vi "DriverFEFY6900.vi"() -> ()   [LabVIEW 2024]
uses:
  <vilib>/Instr/_visa.llb/VISA Set IO Buffer Mask.ctl
  <vilib>/Instr/_visa.llb/VISA Flush IO Buffer Mask.ctl
  <vilib>/Instr/_visa.llb/VISA Configure Serial Port (Instr).vi
panel:
  in  "Parametres":T1
  out "IDnumber":string="COM6"
  in  "Channel A OnOff":bool
  in  "AM FM PM":string[](array[string])=["ChannelB", "Ext VCO - IN"]
  in  "FSK ASK PSK BURS":string[](array[string])=["ChannelB", "Ext AC", "Manual", "Ext DC"]
  out "ChannelB\nChannelBState":bool
  in  "ChannelB OnOff":bool
  in  "Channel B":T2 {"Frequence" min=0.0 max=60000000.0 step=10000000.0 scale=0.0..60000000.0 scale format="%#_6p"; "Phase" scale=0.0..360.0; "DutyCycle" scale=0.0..100.0; "Offset" min=-12.0 max=12.0 step=1.0; "Amplitude" min=0.0 max=24.0 step=1.0}
  out "ChannelAState":bool
  in  "Channel A":T3={"WaveForme"=enum."Sine", "Amplitude"=0.0, "Offset"=0.0, "DutyCycle"=0.0, "Phase"=0.0, "Frequence"=0.0, "Modulation mode"=enum."FSK", "Modulation source"=0, "Trigger Pulse"=0, "FSK frequence"=0, "Manual Sources"=FALSE, " AM modu rate"=0.0, "FM Freq offset"=1000000.0, " PM modu offset"=0.0, "Sweep mode"=enum."Frequency", "Sweep start"=0.0, "Sweep end"=0.0, "Sweep Time (sec)"=0.01, "Type Sweep"=enum."Linear", "Sweep ON/OFF"=FALSE, "Source sweep"=enum."Time", "Incr"=enum."1uHz", "Incr FSK"=enum."1uHz", "Incr Trigger"=enum."1u", "Incr FM"=enum."1uHz"} {"Sweep Time (sec)" min=0.01 max=1000.0 step=1.0 scale=0.0..1000.0; "Sweep end" scale=-12.0..12.0 scale format="%#_6p"; "Sweep start" scale=-12.0..12.0 scale format="%#_6p"; "PM modu offset" min=0.0 max=360.0 step=1.0 scale=0.0..360.0; "FM Freq offset" max=60000000.0 step=1e-06 scale=0.0..60000000.0 scale format="%#_1p"; "AM modu rate" scale=0.0..100.0; "FSK frequence" max=60000000 step=1 scale=0.0..60000000.0 scale format="%.1p"; "Trigger Pulse" max=1048575 step=100 scale=0.0..1048575.0 scale format="%.1p"; "Modulation source" items=["ChannelB", "Ext AC", "Manual", "Ext DC"]; "Frequence" min=0.0 max=60000000.0 step=1e-06 scale=0.0..60000000.0 scale format="%#_6p"; "Phase" scale=0.0..360.0; "DutyCycle" scale=0.0..100.0; "Offset" min=-12.0 max=12.0 step=1.0; "Amplitude" min=0.0 max=24.0 step=1.0}
  out "Com":bool
  in  "PortCOM":string="COM6"
  in  "stop":bool
  in  "Enable Termination\nChar (T)":bool=TRUE
  # "PORT COM"
  # "Sauvegardes et paramètres"
  # "Sweep"
  # "Modulation - Trigger"
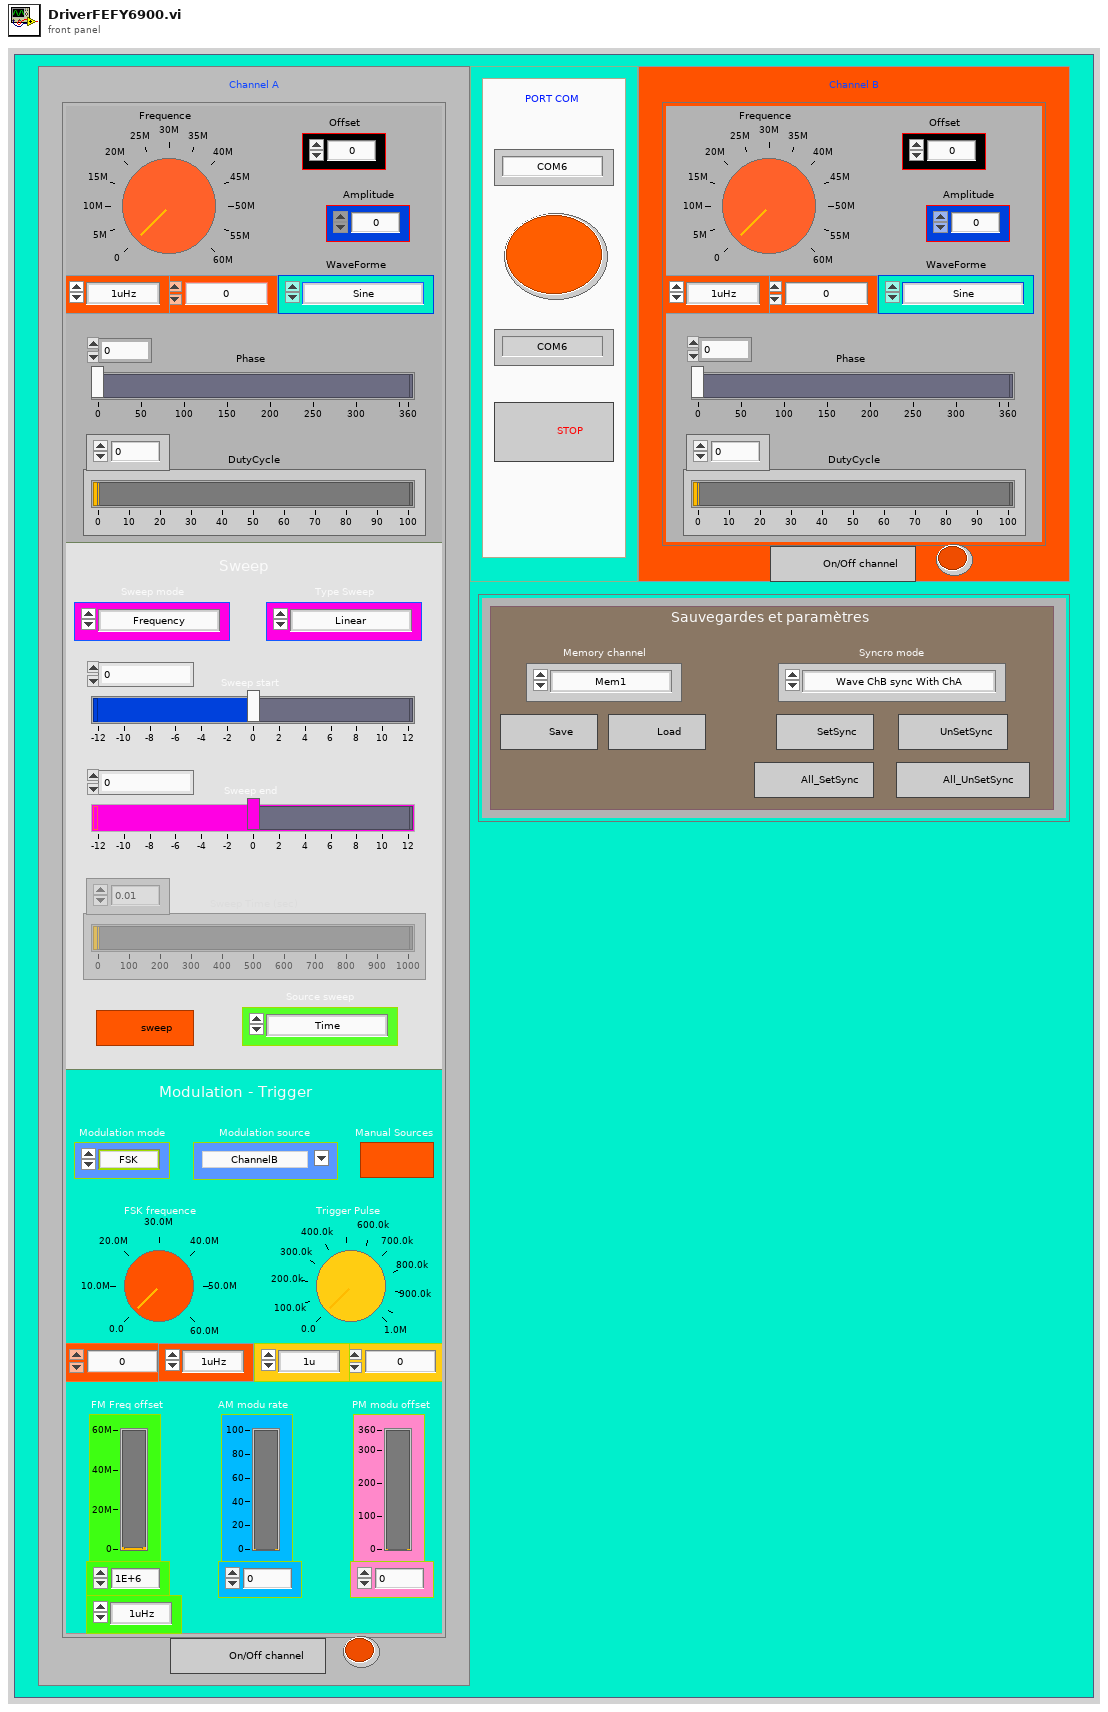
[diagram p1: front panel]
types:
  T1 = cluster{"Memory channel":enum16{"Mem1", "Mem2", "Mem3", "Mem4", "Mem5", "Mem6"}, "Save All param":bool, "Load param":bool, "Syncro mode":enum16{"Wave ChB sync With ChA", "Freq ChB sync With ChA ", "Ampli ChB sync With ChA", "Offset ChB sync With ChA", "DutyC ChB sync With ChA"}, "Set Sync":bool, "UnSet Sync":bool, "All Set Sync":bool, "All UnSet Sync":bool}
  T2 = cluster{"WaveForme":enum16{"Sine", "Square", "Rectangle", "Trapezoid1", "Cmos", "DC", "Triangle", "RAMP", "NegRAMP", "Stair_Triangle", "Stair_Step", "Neg_Stair", "Pos_Exponen", "Neg_Exponen", "P_Fall_Exp", "N_Fall_Exp", "PosLogarit", "NegLogarit", "P_Fall_Log", "N_Fall_Log", "P_Full_Wav", "N_Full_Wav", "P_Half_Wav", "N_Half_Wav", "LorentzPU", "Multitone", "Random_Noise", "ECG", "Trapezoid2", "Sinc_Pulse", "Impulse1", "AWGN", "AM", "FM", "Chrip", "Impulse2", "Arbitraire1", "Arbitraire2"}, "Amplitude":dbl, "Offset":dbl, "DutyCycle":dbl, "Phase":dbl, "Frequence":dbl, "Incr":enum16{"1uHz", "10uHz", "100uHz", "1mHz", "10mHz", "100mHz", "1Hz", "10Hz", "100Hz", "1Khz", "10Khz", "100Khz", "1Mhz", "10Mhz"}}
  T3 = cluster{"WaveForme":enum16{"Sine", "Square", "Rectangle", "Trapezoid1", "Cmos", "ADJ_PULSE", "DC", "Triangle", "RAMP", "NegRAMP", "Stair_Triangle", "Stair_Step", "Neg_Stair", "Pos_Exponen", "Neg_Exponen", "P_Fall_Exp", "N_Fall_Exp", "PosLogarit", "NegLogarit", "P_Fall_Log", "N_Fall_Log", "P_Full_Wav", "N_Full_Wav", "P_Half_Wav", "N_Half_Wav", "LorentzPU", "Multitone", "Random_Noise", "ECG", "Trapezoid2", "Sinc_Pulse", "Impulse1", "AWGN", "AM", "FM", "Chrip", "Impulse2", "Arbitraire1", "Arbitraire2"}, "Amplitude":dbl, "Offset":dbl, "DutyCycle":dbl, "Phase":dbl, "Frequence":dbl, "Modulation mode":enum16{"FSK", "ASK", "PSK", "Burs", "AM", "FM", "PM"}, "Modulation source":u16, "Trigger Pulse":u32, "FSK frequence":u32, "Manual Sources":bool, " AM modu rate":dbl, "FM Freq offset":dbl, " PM modu offset":dbl, "Sweep mode":enum16{"Frequency", "Amplitude", "Offset", "DutyCycle"}, "Sweep start":dbl, "Sweep end":dbl, "Sweep Time (sec)":dbl, "Type Sweep":enum16{"Linear", "Logarithm"}, "Sweep ON/OFF":bool, "Source sweep":enum16{"Time", "VCO IN"}, "Incr":enum16{"1uHz", "10uHz", "100uHz", "1mHz", "10mHz", "100mHz", "1Hz", "10Hz", "100Hz", "1Khz", "10Khz", "100Khz", "1Mhz", "10Mhz"}, "Incr FSK":enum16{"1uHz", "10uHz", "100uHz", "1mHz", "10mHz", "100mHz", "1Hz", "10Hz", "100Hz", "1Khz", "10Khz", "100Khz", "1Mhz", "10Mhz"}, "Incr Trigger":enum16{"1u", "10u", "100u", "1m", "10m", "100m", "1", "10", "100", "1K", "10K", "100K"}, "Incr FM":enum16{"1uHz", "10uHz", "100uHz", "1mHz", "10mHz", "100mHz", "1Hz", "10Hz", "100Hz", "1Khz", "10Khz", "100Khz", "1Mhz", "10Mhz"}}
  T4 = typedef "VISA Set IO Buffer Mask.ctl" = u16
  T5 = enum8{"Enabled", "Disabled", "Disabled and Grayed Out"}
  T6 = enum16{"Sine", "Square", "Rectangle", "Trapezoid1", "Cmos", "ADJ_PULSE", "DC", "Triangle", "RAMP", "NegRAMP", "Stair_Triangle", "Stair_Step", "Neg_Stair", "Pos_Exponen", "Neg_Exponen", "P_Fall_Exp", "N_Fall_Exp", "PosLogarit", "NegLogarit", "P_Fall_Log", "N_Fall_Log", "P_Full_Wav", "N_Full_Wav", "P_Half_Wav", "N_Half_Wav", "LorentzPU", "Multitone", "Random_Noise", "ECG", "Trapezoid2", "Sinc_Pulse", "Impulse1", "AWGN", "AM", "FM", "Chrip", "Impulse2", "Arbitraire1", "Arbitraire2"}
  T7 = typedef "VISA Flush IO Buffer Mask.ctl" = u16
  T8 = enum16{"FSK", "ASK", "PSK", "Burs", "AM", "FM", "PM"}
  T9 = enum16{"Sine", "Square", "Rectangle", "Trapezoid1", "Cmos", "DC", "Triangle", "RAMP", "NegRAMP", "Stair_Triangle", "Stair_Step", "Neg_Stair", "Pos_Exponen", "Neg_Exponen", "P_Fall_Exp", "N_Fall_Exp", "PosLogarit", "NegLogarit", "P_Fall_Log", "N_Fall_Log", "P_Full_Wav", "N_Full_Wav", "P_Half_Wav", "N_Half_Wav", "LorentzPU", "Multitone", "Random_Noise", "ECG", "Trapezoid2", "Sinc_Pulse", "Impulse1", "AWGN", "AM", "FM", "Chrip", "Impulse2", "Arbitraire1", "Arbitraire2"}
  T10 = enum16{"Mem1", "Mem2", "Mem3", "Mem4", "Mem5", "Mem6"}
  T11 = enum16{"Wave ChB sync With ChA", "Freq ChB sync With ChA ", "Ampli ChB sync With ChA", "Offset ChB sync With ChA", "DutyC ChB sync With ChA"}
  T12 = enum16{"Frequency", "Amplitude", "Offset", "DutyCycle"}
  T13 = enum16{"1uHz", "10uHz", "100uHz", "1mHz", "10mHz", "100mHz", "1Hz", "10Hz", "100Hz", "1Khz", "10Khz", "100Khz", "1Mhz", "10Mhz"}
  T14 = enum16{"1u", "10u", "100u", "1m", "10m", "100m", "1", "10", "100", "1K", "10K", "100K"}
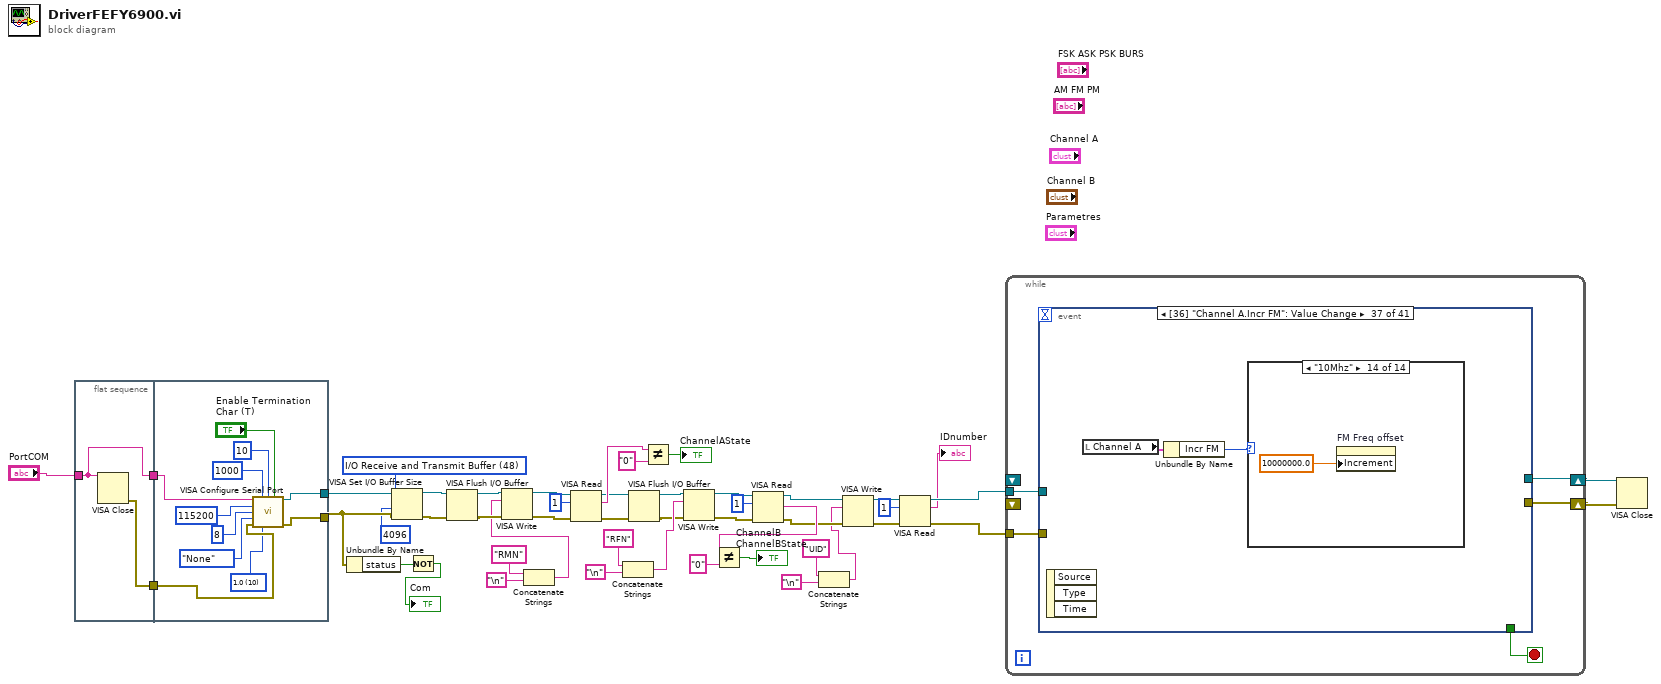
[diagram p0: block diagram]
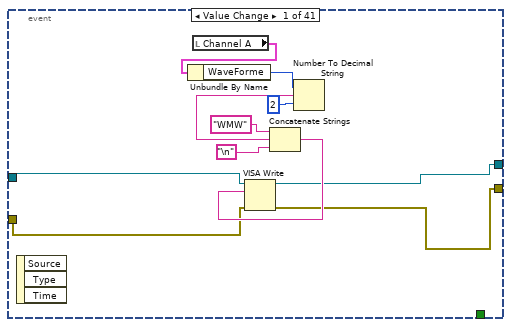
[diagram p2: hidden frame]
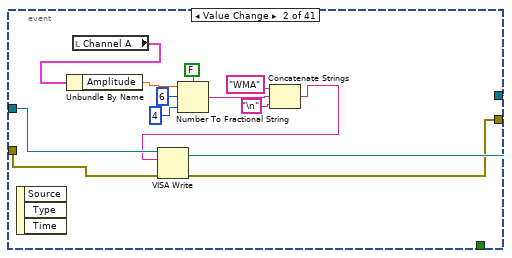
[diagram p3: hidden frame]
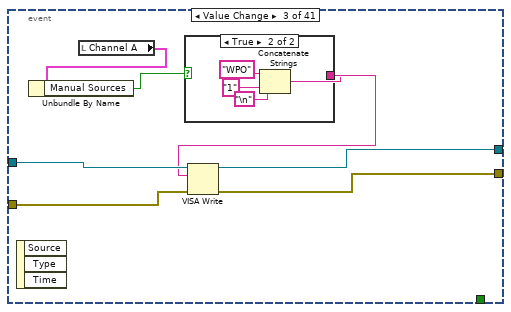
[diagram p4: hidden frame]
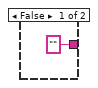
[diagram p5: hidden frame]
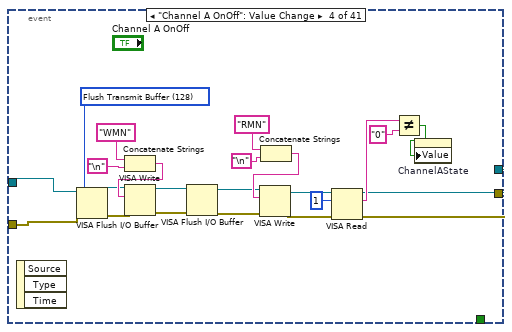
[diagram p6: hidden frame]
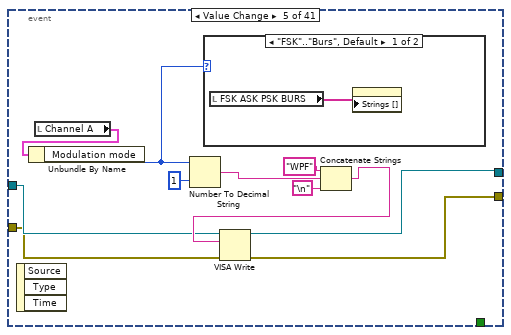
[diagram p7: hidden frame]
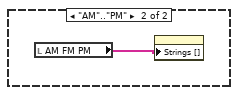
[diagram p8: hidden frame]
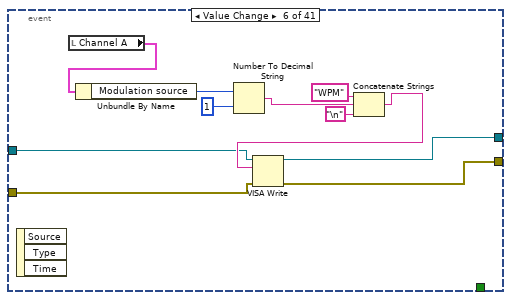
[diagram p9: hidden frame]
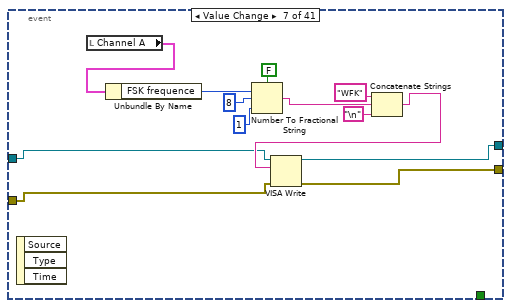
[diagram p10: hidden frame]
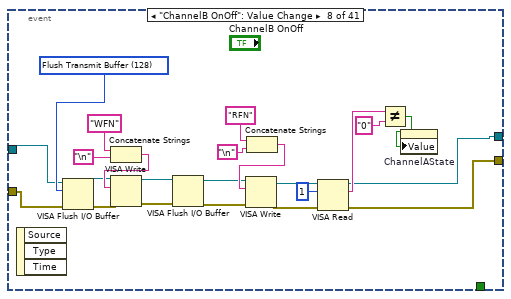
[diagram p11: hidden frame]
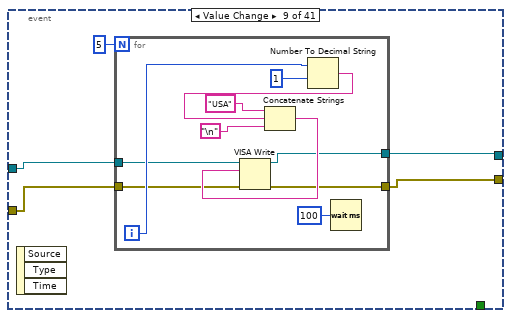
[diagram p12: hidden frame]
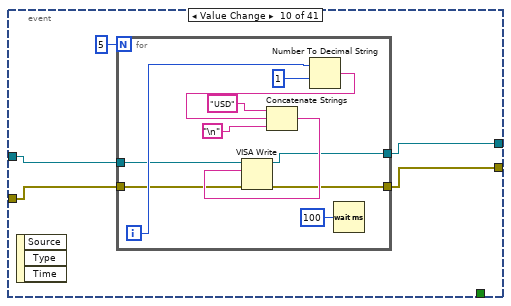
[diagram p13: hidden frame]
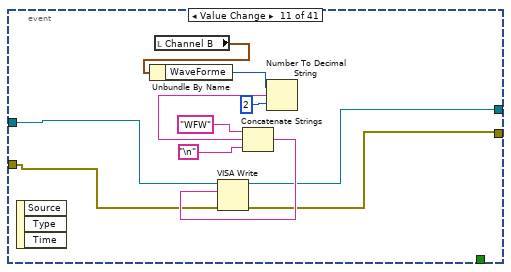
[diagram p14: hidden frame]
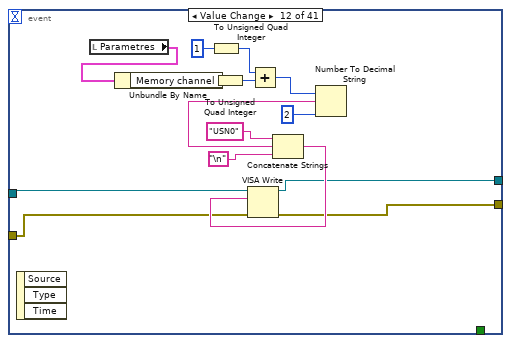
[diagram p15: hidden frame]
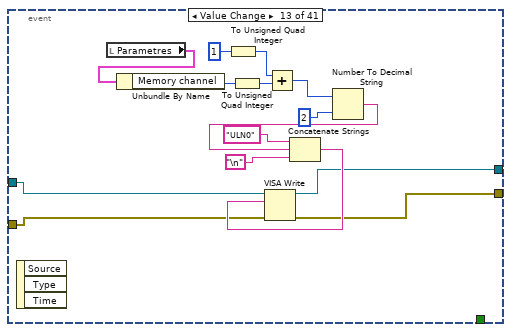
[diagram p16: hidden frame]
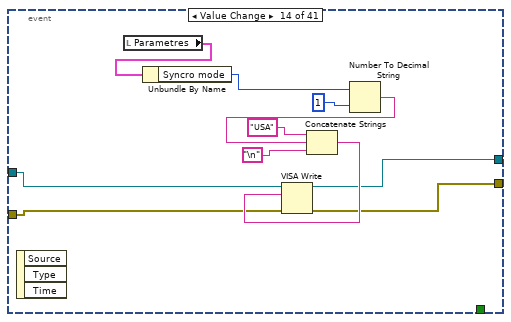
[diagram p17: hidden frame]
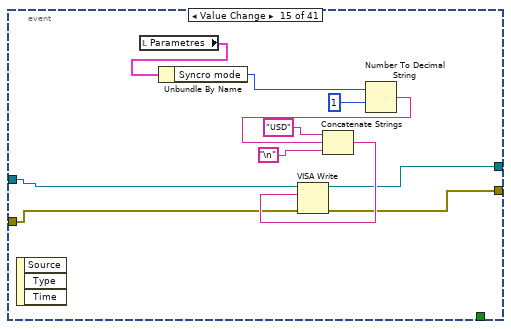
[diagram p18: hidden frame]
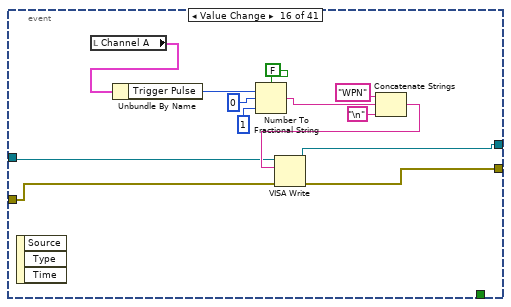
[diagram p19: hidden frame]
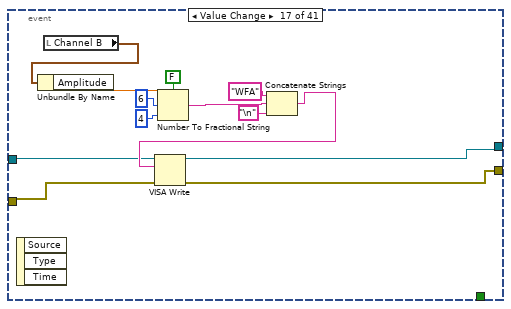
[diagram p20: hidden frame]
diagram:
  w38 = T4 48 items=["I/O Receive Buffer"=16, "I/O Transmit Buffer"=32, "I/O Receive and Transmit Buffer"=48] ("Mask")
  n1 = flat-sequence {
    tunnel: "PortCOM" -> [w50]
    tunnel: [w50] -> w45
    tunnel: [w49] -> w44
    tunnel: w45 -> [w60]
    tunnel: w44 -> [w54]
    tunnel: [w52] -> w41
    tunnel: [w51] -> w40
    frame #0 {
      n2 = VISA Close(VISA resource name=w50) -> (error out=w49:errorcluster)  [unwired: 1 in]
    }
    frame #1 {
      w53 = u16 10 items=["1.0"=10, "1.5"=15, "2.0"=20] ("stop bits (10: 1 bit)")
      n3 = call-poly "VISA Configure Serial Port"("VISA resource name"=w60, "timeout (10sec)"=u32 1000, "termination char\n(0xA = '\\n' = LF)"=u8 10 ("termination char\n(0xA = '\\n' = LF)"), "Enable Termination\nChar (T)"="Enable Termination\nChar (T)", "baud rate (9600)"=u32 115200, "data bits (8)"=u16 8, "parity (0:none)"=enum16{"None", "Odd", "Even", "Mark", "Space"}."None", "error in (no error)"=w54, "stop bits (10: 1 bit)"=w53) -> ("VISA resource name out"=w52:refnum<visa-resource-name>, "error out"=w51:errorcluster)  [unwired: 5 in]
    }
  }
  n4 = Unbundle By Name(w40) -> ("status"=w43:bool)
  n5 = VISA Set I/O Buffer Size(VISA resource name=w41, mask (16)=w38, size (4096)=u32 4096, error in (no error)=w40) -> (VISA resource name out=w31:refnum<visa-resource-name>, error out=w32:errorcluster)
  n6 = Not(x=w43) -> (.not. x?=→"Com":bool)
  n7 = VISA Flush I/O Buffer(VISA resource name=w31, error in (no error)=w32) -> (VISA resource name out=w36:refnum<visa-resource-name>, error out=w37:errorcluster)  [unwired: 1 in]
  n8 = Concatenate Strings("RMN" ("string"), "\n") -> (w33:string)
  n9 = VISA Write(VISA resource name=w36, write buffer=w33, error in (no error)=w37) -> (VISA resource name out=w34:refnum<visa-resource-name>, error out=w35:errorcluster)  [unwired: 1 out]
  n10 = VISA Read(VISA resource name=w34, byte count=u32 1, error in (no error)=w35) -> (VISA resource name out=w17:refnum<visa-resource-name>, read buffer=w27:string, error out=w16:errorcluster)  [unwired: 1 out]
  n11 = Concatenate Strings("RFN" ("string"), "\n") -> (w22:string)
  n12 = VISA Flush I/O Buffer(VISA resource name=w17, error in (no error)=w16) -> (VISA resource name out=w19:refnum<visa-resource-name>, error out=w18:errorcluster)  [unwired: 1 in]
  n13 = Not Equal?(x=w27, y="0" ("x")) -> (x != y?=→"ChannelAState":bool)
  n14 = VISA Write(VISA resource name=w19, write buffer=w22, error in (no error)=w18) -> (VISA resource name out=w21:refnum<visa-resource-name>, error out=w20:errorcluster)  [unwired: 1 out]
  n15 = VISA Read(VISA resource name=w21, byte count=u32 1, error in (no error)=w20) -> (VISA resource name out=w11:refnum<visa-resource-name>, read buffer=w14:string, error out=w10:errorcluster)  [unwired: 1 out]
  n16 = Not Equal?(x=w14, y="0" ("x")) -> (x != y?=→"ChannelB\nChannelBState":bool)
  n17 = Concatenate Strings("UID" ("string"), "\n") -> (w7:string)
  n18 = VISA Write(VISA resource name=w11, write buffer=w7, error in (no error)=w10) -> (VISA resource name out=w6:refnum<visa-resource-name>, error out=w5:errorcluster)  [unwired: 1 out]
  n19 = VISA Read(VISA resource name=w6, byte count=u32 1, error in (no error)=w5) -> (VISA resource name out=w3:refnum<visa-resource-name>, read buffer=→"IDnumber":string, error out=w2:errorcluster)  [unwired: 1 out]
  n20 = while {
    shift-right: [w66] -> w48
    shift-left: _ -> [_]
    shift-right: [w64] -> w47
    shift-left: _ -> [_]
    tunnel: w2 -> [w63]
    tunnel: w3 -> [w62]
    stop <- w65 stop-if-true
    n21 = event shown="[36] \"Channel A.Incr FM\": Value Change" {
      selector: _ -> [_ _ _ _ _ _ _ _ _ _ _ _ _ _ _ _ _ _ _ _ _ _ _ _ _ _ _ _ _ _ _ _ _ _ _ _ _ _ _ _ _]
      dyn-events: _ -> [_ _ _ _ _ _ _ _ _ _ _ _ _ _ _ _ _ _ _ _ _ _ _ _ _ _ _ _ _ _ _ _ _ _ _ _ _ _ _ _ _]
      timeout: _ -> [_ _ _ _ _ _ _ _ _ _ _ _ _ _ _ _ _ _ _ _ _ _ _ _ _ _ _ _ _ _ _ _ _ _ _ _ _ _ _ _ _]
      tunnel: w63 -> [w76 w88 w94 w111 w131 w139 w154 w163 w188 w204 w220 w237 w246 w262 w272 w283 w301 w311 w325 w335 w351 w362 w374 w387 w402 w414 w424 w439 w464 w498 w537 w555 _ _ _ _ _ w645 w658 w661 w674]
      tunnel: [w75 w86 w91 _ w129 w141 w152 w165 w186 w202 w218 w235 w244 w260 w270 w281 w299 w309 w323 w333 w349 w360 w372 w385 w400 w411 w422 w437 w462 w496 _ _ _ _ _ _ _ w643 w656 w661 w672] -> _
      tunnel: w62 -> [w74 w89 w95 w112 w132 w140 w155 w164 w189 w205 w221 w238 w247 w263 w273 w284 w302 w312 w326 w336 w352 w363 w375 w388 w403 w413 w425 w440 w463 w499 w538 w556 _ _ _ _ _ w646 w659 w662 w675]
      tunnel: [w73 w87 w96 w105 w130 w142 w153 w166 w187 w203 w219 w236 w245 w261 w271 w282 w300 w310 w324 w334 w350 w361 w373 w386 w401 w412 w423 w438 w461 w497 w536 w554 _ _ _ _ _ w644 w657 w662 w673] -> w66
      tunnel: [_ _ _ _ _ _ _ _ _ _ _ _ _ _ _ _ _ _ _ _ _ _ _ _ _ _ _ _ _ _ _ _ _ _ _ _ _ _ _ "stop" _] -> w65
      tunnel: [_ _ _ w104 _ _ _ _ _ _ _ _ _ _ _ _ _ _ _ _ _ _ _ _ _ _ _ _ _ _ w535 w553 _ _ _ _ _ _ _ _ _] -> w64
      event "Channel A.WaveForme": Value Change {
        n22 = event-data() -> ()  [unwired: 1 in, 3 out]
        n23 = local read "Channel A"() -> (w68:T3)
        n24 = Unbundle By Name(w68) -> ("WaveForme"=w67:T6)
        n25 = Number To Decimal String(number=w67, width (-)=i16 2) -> (decimal integer string=w71:string)
        n26 = Concatenate Strings("WMW" ("write buffer"), w71, "\n") -> (w77:string)
        n27 = VISA Write(VISA resource name=w74, write buffer=w77, error in (no error)=w76) -> (VISA resource name out=w73:refnum<visa-resource-name>, error out=w75:errorcluster)  [unwired: 1 out]
      }
      event "Channel A.Amplitude": Value Change {
        n28 = event-data() -> ()  [unwired: 1 in, 3 out]
        n29 = local read "Channel A"() -> (w90:T3)
        n30 = Unbundle By Name(w90) -> ("Amplitude"=w82:dbl)
        n31 = Number To Fractional String(use system decimal point (T)=FALSE, number=w82, width (-)=i16 6, precision (6)=i16 4 ("width (-)")) -> (F-format string=w80:string)
        n32 = Concatenate Strings("WMA" ("string"), w80, "\n") -> (w84:string)
        n33 = VISA Write(VISA resource name=w89, write buffer=w84, error in (no error)=w88) -> (VISA resource name out=w87:refnum<visa-resource-name>, error out=w86:errorcluster)  [unwired: 1 out]
      }
      event "Channel A.Manual Sources": Value Change {
        n34 = event-data() -> ()  [unwired: 1 in, 3 out]
        n35 = local read "Channel A"() -> (w97:T3)
        n36 = Unbundle By Name(w97) -> ("Manual Sources"=w92:bool)
        n37 = case shown="True" w92 {
          tunnel: ["" w100] -> w93
          frame False {
          }
          frame True {
            n38 = Concatenate Strings("WPO" ("string"), "1" ("string"), "\n") -> (w100:string)
          }
        }
        n39 = VISA Write(VISA resource name=w95, write buffer=w93, error in (no error)=w94) -> (VISA resource name out=w96:refnum<visa-resource-name>, error out=w91:errorcluster)  [unwired: 1 out]
      }
      event "Channel A OnOff": Value Change {
        w114 = T7 128 items=["Flush Receive Buffer"=16, "Write Transmit Buffer to Device"=32, "Flush Receive Buffer (No I/O)"=64, "Flush Transmit Buffer"=128] ("Mask")
        n40 = event-data() -> ()  [unwired: 1 in, 3 out]
        n41 = VISA Flush I/O Buffer(VISA resource name=w112, mask (16)=w114, error in (no error)=w111) -> (VISA resource name out=w115:refnum<visa-resource-name>, error out=w119:errorcluster)
        n42 = Concatenate Strings("WMN" ("string"), "\n") -> (w118:string)
        n43 = VISA Write(VISA resource name=w115, write buffer=w118, error in (no error)=w119) -> (VISA resource name out=w113:refnum<visa-resource-name>, error out=w120:errorcluster)  [unwired: 1 out]
        n44 = VISA Flush I/O Buffer(VISA resource name=w113, error in (no error)=w120) -> (VISA resource name out=w123:refnum<visa-resource-name>, error out=w122:errorcluster)  [unwired: 1 in]
        n45 = Concatenate Strings("RMN" ("string"), "\n") -> (w125:string)
        n46 = VISA Write(VISA resource name=w123, write buffer=w125, error in (no error)=w122) -> (VISA resource name out=w107:refnum<visa-resource-name>, error out=w106:errorcluster)  [unwired: 1 out]
        n47 = VISA Read(VISA resource name=w107, byte count=u32 1, error in (no error)=w106) -> (VISA resource name out=w105:refnum<visa-resource-name>, read buffer=w110:string, error out=w104:errorcluster)  [unwired: 1 out]
        n48 = Not Equal?(x=w110, y="0") -> (x != y?=w108:bool)
        n49 = property on="ChannelAState" class="Bool (strict)"("Value"=w108) -> ()  [unwired: 2 in, 2 out]
      }
      event "Channel A.Modulation mode": Value Change {
        n50 = event-data() -> ()  [unwired: 1 in, 3 out]
        n51 = local read "Channel A"() -> (w136:T3)
        n52 = Unbundle By Name(w136) -> ("Modulation mode"=w126:T8)
        n53 = Number To Decimal String(number=w126, width (-)=i16 1) -> (decimal integer string=w127:string)
        n54 = case shown="\"FSK\"..\"Burs\", Default" w126 {
          frame "FSK".."Burs", Default {
            n55 = local read "FSK ASK PSK BURS"() -> (w137:string[])
            n56 = property on="Modulation source" class="Ring (strict)"("Strings []"=w137) -> ()  [unwired: 2 in, 2 out]
          }
          frame "AM".."PM" {
            n57 = local read "AM FM PM"() -> (w138:string[])
            n58 = property on="Modulation source" class="Ring (strict)"("Strings []"=w138) -> ()  [unwired: 2 in, 2 out]
          }
        }
        n59 = Concatenate Strings("WPF" ("string"), w127, "\n") -> (w135:string)
        n60 = VISA Write(VISA resource name=w132, write buffer=w135, error in (no error)=w131) -> (VISA resource name out=w130:refnum<visa-resource-name>, error out=w129:errorcluster)  [unwired: 1 out]
      }
      event "Channel A.Modulation source": Value Change {
        n61 = event-data() -> ()  [unwired: 1 in, 3 out]
        n62 = local read "Channel A"() -> (w149:T3)
        n63 = Unbundle By Name(w149) -> ("Modulation source"=w147:u16)
        n64 = Number To Decimal String(number=w147, width (-)=i16 1) -> (decimal integer string=w146:string)
        n65 = Concatenate Strings("WPM" ("string"), w146, "\n") -> (w148:string)
        n66 = VISA Write(VISA resource name=w140, write buffer=w148, error in (no error)=w139) -> (VISA resource name out=w142:refnum<visa-resource-name>, error out=w141:errorcluster)  [unwired: 1 out]
      }
      event "Channel A.FSK frequence": Value Change {
        n67 = event-data() -> ()  [unwired: 1 in, 3 out]
        n68 = local read "Channel A"() -> (w162:T3)
        n69 = Unbundle By Name(w162) -> ("FSK frequence"=w160:u32)
        n70 = Number To Fractional String(use system decimal point (T)=FALSE, number=w160, width (-)=i16 8, precision (6)=i16 1 ("width (-)")) -> (F-format string=w159:string)
        n71 = Concatenate Strings("WFK" ("string"), w159, "\n") -> (w161:string)
        n72 = VISA Write(VISA resource name=w155, write buffer=w161, error in (no error)=w154) -> (VISA resource name out=w153:refnum<visa-resource-name>, error out=w152:errorcluster)  [unwired: 1 out]
      }
      event "ChannelB OnOff": Value Change {
        w169 = T7 128 items=["Flush Receive Buffer"=16, "Write Transmit Buffer to Device"=32, "Flush Receive Buffer (No I/O)"=64, "Flush Transmit Buffer"=128] ("Mask")
        n73 = event-data() -> ()  [unwired: 1 in, 3 out]
        n74 = VISA Flush I/O Buffer(VISA resource name=w164, mask (16)=w169, error in (no error)=w163) -> (VISA resource name out=w179:refnum<visa-resource-name>, error out=w181:errorcluster)
        n75 = Concatenate Strings("WFN" ("string"), "\n") -> (w180:string)
        n76 = VISA Write(VISA resource name=w179, write buffer=w180, error in (no error)=w181) -> (VISA resource name out=w178:refnum<visa-resource-name>, error out=w182:errorcluster)  [unwired: 1 out]
        n77 = VISA Flush I/O Buffer(VISA resource name=w178, error in (no error)=w182) -> (VISA resource name out=w184:refnum<visa-resource-name>, error out=w183:errorcluster)  [unwired: 1 in]
        n78 = Concatenate Strings("RFN" ("string"), "\n") -> (w185:string)
        n79 = VISA Write(VISA resource name=w184, write buffer=w185, error in (no error)=w183) -> (VISA resource name out=w175:refnum<visa-resource-name>, error out=w174:errorcluster)  [unwired: 1 out]
        n80 = VISA Read(VISA resource name=w175, byte count=u32 1, error in (no error)=w174) -> (VISA resource name out=w166:refnum<visa-resource-name>, read buffer=w177:string, error out=w165:errorcluster)  [unwired: 1 out]
        n81 = Not Equal?(x=w177, y="0") -> (x != y?=w176:bool)
        n82 = property on="ChannelAState" class="Bool (strict)"("Value"=w176) -> ()  [unwired: 2 in, 2 out]
      }
      event "Parametres.All Set Sync": Value Change {
        n83 = event-data() -> ()  [unwired: 1 in, 3 out]
        n84 = for {
          N: 5 -> [_]
          tunnel: w189 -> [w195]
          tunnel: w188 -> [w194]
          tunnel: [w193] -> w187
          tunnel: [w192] -> w186
          i -> [w196]
          n85 = Number To Decimal String(number=w196, width (-)=i16 1) -> (decimal integer string=w200:string)
          n86 = Concatenate Strings("USA" ("write buffer"), w200, "\n") -> (w201:string)
          n87 = VISA Write(VISA resource name=w195, write buffer=w201, error in (no error)=w194) -> (VISA resource name out=w193:refnum<visa-resource-name>, error out=w192:errorcluster)  [unwired: 1 out]
          n88 = Wait (ms)(milliseconds to wait=u32 100) -> ()  [unwired: 1 out]
        }
      }
      event "Parametres.All UnSet Sync": Value Change {
        n89 = event-data() -> ()  [unwired: 1 in, 3 out]
        n90 = for {
          N: 5 -> [_]
          tunnel: w205 -> [w211]
          tunnel: w204 -> [w210]
          tunnel: [w209] -> w203
          tunnel: [w208] -> w202
          i -> [w212]
          n91 = Number To Decimal String(number=w212, width (-)=i16 1) -> (decimal integer string=w216:string)
          n92 = Concatenate Strings("USD" ("write buffer"), w216, "\n") -> (w217:string)
          n93 = VISA Write(VISA resource name=w211, write buffer=w217, error in (no error)=w210) -> (VISA resource name out=w209:refnum<visa-resource-name>, error out=w208:errorcluster)  [unwired: 1 out]
          n94 = Wait (ms)(milliseconds to wait=u32 100) -> ()  [unwired: 1 out]
        }
      }
      event "Channel B.WaveForme": Value Change {
        n95 = event-data() -> ()  [unwired: 1 in, 3 out]
        n96 = local read "Channel B"() -> (w223:T2)
        n97 = Unbundle By Name(w223) -> ("WaveForme"=w222:T9)
        n98 = Number To Decimal String(number=w222, width (-)=i16 2) -> (decimal integer string=w226:string)
        n99 = Concatenate Strings("WFW" ("write buffer"), w226, "\n") -> (w228:string)
        n100 = VISA Write(VISA resource name=w221, write buffer=w228, error in (no error)=w220) -> (VISA resource name out=w219:refnum<visa-resource-name>, error out=w218:errorcluster)  [unwired: 1 out]
      }
      event "Parametres.Save All param": Value Change {
        n101 = event-data() -> ()  [unwired: 1 in, 3 out]
        n102 = local read "Parametres"() -> (w234:T1)
        n103 = Unbundle By Name(w234) -> ("Memory channel"=w233:T10)
        n104 = To Unsigned Quad Integer(1:1) -> (0:w229:u64)
        n105 = To Unsigned Quad Integer(1:w233) -> (0:w230:u64)
        n106 = Add(x=w229, y=w230) -> (x+y=w231:u64)
        n107 = Number To Decimal String(number=w231, width (-)=i16 2) -> (decimal integer string=w242:string)
        n108 = Concatenate Strings("USN0" ("write buffer"), w242, "\n") -> (w243:string)
        n109 = VISA Write(VISA resource name=w238, write buffer=w243, error in (no error)=w237) -> (VISA resource name out=w236:refnum<visa-resource-name>, error out=w235:errorcluster)  [unwired: 1 out]
      }
      event "Parametres.Load param": Value Change {
        n110 = event-data() -> ()  [unwired: 1 in, 3 out]
        n111 = local read "Parametres"() -> (w256:T1)
        n112 = Unbundle By Name(w256) -> ("Memory channel"=w255:T10)
        n113 = To Unsigned Quad Integer(1:1) -> (0:w252:u64)
        n114 = To Unsigned Quad Integer(1:w255) -> (0:w253:u64)
        n115 = Add(x=w252, y=w253) -> (x+y=w254:u64)
        n116 = Number To Decimal String(number=w254, width (-)=i16 2) -> (decimal integer string=w257:string)
        n117 = Concatenate Strings("ULN0" ("write buffer"), w257, "\n") -> (w258:string)
        n118 = VISA Write(VISA resource name=w247, write buffer=w258, error in (no error)=w246) -> (VISA resource name out=w245:refnum<visa-resource-name>, error out=w244:errorcluster)  [unwired: 1 out]
      }
      event "Parametres.Set Sync": Value Change {
        n119 = event-data() -> ()  [unwired: 1 in, 3 out]
        n120 = local read "Parametres"() -> (w267:T1)
        n121 = Unbundle By Name(w267) -> ("Syncro mode"=w259:T11)
        n122 = Number To Decimal String(number=w259, width (-)=i16 1) -> (decimal integer string=w268:string)
        n123 = Concatenate Strings("USA" ("write buffer"), w268, "\n") -> (w269:string)
        n124 = VISA Write(VISA resource name=w263, write buffer=w269, error in (no error)=w262) -> (VISA resource name out=w261:refnum<visa-resource-name>, error out=w260:errorcluster)  [unwired: 1 out]
      }
      event "Parametres.UnSet Sync": Value Change {
        n125 = event-data() -> ()  [unwired: 1 in, 3 out]
        n126 = local read "Parametres"() -> (w278:T1)
        n127 = Unbundle By Name(w278) -> ("Syncro mode"=w277:T11)
        n128 = Number To Decimal String(number=w277, width (-)=i16 1) -> (decimal integer string=w279:string)
        n129 = Concatenate Strings("USD" ("write buffer"), w279, "\n") -> (w280:string)
        n130 = VISA Write(VISA resource name=w273, write buffer=w280, error in (no error)=w272) -> (VISA resource name out=w271:refnum<visa-resource-name>, error out=w270:errorcluster)  [unwired: 1 out]
      }
      event "Channel A.Trigger Pulse": Value Change {
        n131 = event-data() -> ()  [unwired: 1 in, 3 out]
        n132 = local read "Channel A"() -> (w293:T3)
        n133 = Unbundle By Name(w293) -> ("Trigger Pulse"=w291:u32)
        n134 = Number To Fractional String(use system decimal point (T)=FALSE, number=w291, width (-)=i16 0, precision (6)=i16 1 ("width (-)")) -> (F-format string=w290:string)
        n135 = Concatenate Strings("WPN" ("string"), w290, "\n") -> (w292:string)
        n136 = VISA Write(VISA resource name=w284, write buffer=w292, error in (no error)=w283) -> (VISA resource name out=w282:refnum<visa-resource-name>, error out=w281:errorcluster)  [unwired: 1 out]
      }
      event "Channel B.Amplitude": Value Change {
        n137 = event-data() -> ()  [unwired: 1 in, 3 out]
        n138 = local read "Channel B"() -> (w303:T2)
        n139 = Unbundle By Name(w303) -> ("Amplitude"=w298:dbl)
        n140 = Number To Fractional String(use system decimal point (T)=FALSE, number=w298, width (-)=i16 6, precision (6)=i16 4) -> (F-format string=w294:string)
        n141 = Concatenate Strings("WFA" ("string"), w294, "\n") -> (w306:string)
        n142 = VISA Write(VISA resource name=w302, write buffer=w306, error in (no error)=w301) -> (VISA resource name out=w300:refnum<visa-resource-name>, error out=w299:errorcluster)  [unwired: 1 out]
      }
      event "Channel B.Offset": Value Change {
        n143 = event-data() -> ()  [unwired: 1 in, 3 out]
        n144 = local read "Channel B"() -> (w319:T2)
        n145 = Unbundle By Name(w319) -> ("Offset"=w317:dbl)
        n146 = Number To Fractional String(use system decimal point (T)=FALSE, number=w317, width (-)=i16 6, precision (6)=i16 3 ("width (-)")) -> (F-format string=w316:string)
        n147 = Concatenate Strings("WFO" ("string"), w316, "\n") -> (w318:string)
        n148 = VISA Write(VISA resource name=w312, write buffer=w318, error in (no error)=w311) -> (VISA resource name out=w310:refnum<visa-resource-name>, error out=w309:errorcluster)  [unwired: 1 out]
      }
      event "Channel B.DutyCycle": Value Change {
        n149 = event-data() -> ()  [unwired: 1 in, 3 out]
        n150 = local read "Channel B"() -> (w332:T2)
        n151 = Unbundle By Name(w332) -> ("DutyCycle"=w330:dbl)
        n152 = Number To Fractional String(use system decimal point (T)=FALSE, number=w330, width (-)=i16 6, precision (6)=i16 3) -> (F-format string=w329:string)
        n153 = Concatenate Strings("WFD" ("string"), w329, "\n") -> (w331:string)
        n154 = VISA Write(VISA resource name=w326, write buffer=w331, error in (no error)=w325) -> (VISA resource name out=w324:refnum<visa-resource-name>, error out=w323:errorcluster)  [unwired: 1 out]
      }
      event "Channel A.AM modu rate": Value Change {
        n155 = event-data() -> ()  [unwired: 1 in, 3 out]
        n156 = local read "Channel A"() -> (w345:T3)
        n157 = Unbundle By Name(w345) -> ("AM modu rate"=w343:dbl)
        n158 = Number To Fractional String(use system decimal point (T)=FALSE, number=w343, width (-)=i16 4, precision (6)=i16 1) -> (F-format string=w342:string)
        n159 = Concatenate Strings("WPR" ("string"), w342, "\n") -> (w344:string)
        n160 = VISA Write(VISA resource name=w336, write buffer=w344, error in (no error)=w335) -> (VISA resource name out=w334:refnum<visa-resource-name>, error out=w333:errorcluster)  [unwired: 1 out]
      }
      event "Channel B.Phase": Value Change {
        n161 = event-data() -> ()  [unwired: 1 in, 3 out]
        n162 = local read "Channel B"() -> (w358:T2)
        n163 = Unbundle By Name(w358) -> ("Phase"=w356:dbl)
        n164 = Number To Fractional String(use system decimal point (T)=FALSE, number=w356, width (-)=i16 6, precision (6)=i16 3) -> (F-format string=w355:string)
        n165 = Concatenate Strings("WFP" ("string"), w355, "\n") -> (w357:string)
        n166 = VISA Write(VISA resource name=w352, write buffer=w357, error in (no error)=w351) -> (VISA resource name out=w350:refnum<visa-resource-name>, error out=w349:errorcluster)  [unwired: 1 out]
      }
      event "Channel A.FM Freq offset": Value Change {
        n167 = event-data() -> ()  [unwired: 1 in, 3 out]
        n168 = local read "Channel A"() -> (w371:T3)
        n169 = Unbundle By Name(w371) -> ("FM Freq offset"=w369:dbl)
        n170 = Number To Fractional String(use system decimal point (T)=FALSE, number=w369, width (-)=i16 0, precision (6)=i16 6) -> (F-format string=w359:string)
        n171 = Concatenate Strings("WFM" ("string"), w359, "\n") -> (w370:string)
        n172 = VISA Write(VISA resource name=w363, write buffer=w370, error in (no error)=w362) -> (VISA resource name out=w361:refnum<visa-resource-name>, error out=w360:errorcluster)  [unwired: 1 out]
      }
      event "Channel A.PM modu offset": Value Change {
        n173 = event-data() -> ()  [unwired: 1 in, 3 out]
        n174 = local read "Channel A"() -> (w384:T3)
        n175 = Unbundle By Name(w384) -> ("PM modu offset"=w382:dbl)
        n176 = Number To Fractional String(use system decimal point (T)=FALSE, number=w382, width (-)=i16 9, precision (6)=i16 1) -> (F-format string=w381:string)
        n177 = Concatenate Strings("WPP" ("string"), w381, "\n") -> (w383:string)
        n178 = VISA Write(VISA resource name=w375, write buffer=w383, error in (no error)=w374) -> (VISA resource name out=w373:refnum<visa-resource-name>, error out=w372:errorcluster)  [unwired: 1 out]
      }
      event "Channel A.Sweep Time (sec)": Value Change {
        n179 = event-data() -> ()  [unwired: 1 in, 3 out]
        n180 = local read "Channel A"() -> (w397:T3)
        n181 = Unbundle By Name(w397) -> ("Sweep Time (sec)"=w395:dbl)
        n182 = Number To Fractional String(use system decimal point (T)=FALSE, number=w395, width (-)=i16 5, precision (6)=i16 2) -> (F-format string=w394:string)
        n183 = Concatenate Strings("STI" ("string"), w394, "\n") -> (w396:string)
        n184 = VISA Write(VISA resource name=w388, write buffer=w396, error in (no error)=w387) -> (VISA resource name out=w386:refnum<visa-resource-name>, error out=w385:errorcluster)  [unwired: 1 out]
      }
      event "Channel A.Type Sweep": Value Change {
        n185 = event-data() -> ()  [unwired: 1 in, 3 out]
        n186 = local read "Channel A"() -> (w408:T3)
        n187 = Unbundle By Name(w408) -> ("Type Sweep"=w398:enum16{"Linear", "Logarithm"})
        n188 = Number To Decimal String(number=w398, width (-)=i16 1 ("precision (6)")) -> (decimal integer string=w406:string)
        n189 = Concatenate Strings("SMO" ("string"), w406, "\n") -> (w407:string)
        n190 = VISA Write(VISA resource name=w403, write buffer=w407, error in (no error)=w402) -> (VISA resource name out=w401:refnum<visa-resource-name>, error out=w400:errorcluster)  [unwired: 1 out]
      }
      event "Channel A.Sweep ON/OFF": Value Change {
        n191 = event-data() -> ()  [unwired: 1 in, 3 out]
        n192 = local read "Channel A"() -> (w420:T3)
        n193 = Unbundle By Name(w420) -> ("Sweep ON/OFF"=w410:bool)
        n194 = Boolean To (0,1)(Boolean=w410) -> (0, 1=w409:i16)
        n195 = Number To Decimal String(number=w409, width (-)=i16 1 ("precision (6)")) -> (decimal integer string=w418:string)
        n196 = Concatenate Strings("SBE" ("string"), w418, "\n") -> (w419:string)
        n197 = VISA Write(VISA resource name=w413, write buffer=w419, error in (no error)=w414) -> (VISA resource name out=w412:refnum<visa-resource-name>, error out=w411:errorcluster)  [unwired: 1 out]
      }
      event "Channel A.Source sweep": Value Change {
        n198 = event-data() -> ()  [unwired: 1 in, 3 out]
        n199 = local read "Channel A"() -> (w431:T3)
        n200 = Unbundle By Name(w431) -> ("Source sweep"=w421:enum16{"Time", "VCO IN"})
        n201 = Number To Decimal String(number=w421, width (-)=i16 1 ("precision (6)")) -> (decimal integer string=w429:string)
        n202 = Concatenate Strings("SXY" ("string"), w429, "\n") -> (w430:string)
        n203 = case shown="\"Time\", Default" w421 {
          frame "Time", Default {
            n204 = property on="Sweep Time (sec)" class="Slide (strict)"("DisabledEnum"=T5."Enabled" ("Disabled")) -> ()  [unwired: 2 in, 2 out]
          }
          frame "VCO IN" {
            n205 = property on="Sweep Time (sec)" class="Slide (strict)"("DisabledEnum"=T5."Disabled and Grayed Out" ("Disabled")) -> ()  [unwired: 2 in, 2 out]
          }
        }
        n206 = VISA Write(VISA resource name=w425, write buffer=w430, error in (no error)=w424) -> (VISA resource name out=w423:refnum<visa-resource-name>, error out=w422:errorcluster)  [unwired: 1 out]
      }
      event "Channel A.Sweep mode": Value Change {
        n207 = event-data() -> ()  [unwired: 1 in, 3 out]
        n208 = local read "Channel A"() -> (w436:T3)
        n209 = Unbundle By Name(w436) -> ("Sweep mode"=w434:T12)
        n210 = Number To Decimal String(number=w434, width (-)=i16 1) -> (decimal integer string=w443:string)
        n211 = Concatenate Strings("SOB" ("write buffer"), w443, "\n") -> (w444:string)
        n212 = VISA Write(VISA resource name=w440, write buffer=w444, error in (no error)=w439) -> (VISA resource name out=w438:refnum<visa-resource-name>, error out=w437:errorcluster)  [unwired: 1 out]
        n213 = case shown="\"Offset\"" w434 {
          frame "Frequency", Default {
            n214 = property on="Sweep start" class="Slide (strict)"("Scale.Minimum"=0.0 ("Scale.Range:Maximum")) -> ()  [unwired: 2 in, 2 out]
            n215 = property on="Sweep end" class="Slide (strict)"("Scale.Minimum"=0.0 ("Scale.Range:Maximum")) -> ()  [unwired: 2 in, 2 out]
            n216 = property on="Sweep start" class="Slide (strict)"("Scale.Maximum"=10000000.0 ("Scale.Range:Maximum")) -> ()  [unwired: 2 in, 2 out]
            n217 = property on="Sweep end" class="Slide (strict)"("Scale.Maximum"=10000000.0 ("Scale.Range:Maximum")) -> ()  [unwired: 2 in, 2 out]
          }
          frame "Offset" {
            n218 = property on="Sweep start" class="Slide (strict)"("Scale.Minimum"=-12.0 ("Scale.Range:Maximum")) -> ()  [unwired: 2 in, 2 out]
            n219 = property on="Sweep start" class="Slide (strict)"("Scale.Maximum"=12.0 ("Scale.Range:Maximum")) -> ()  [unwired: 2 in, 2 out]
            n220 = property on="Sweep end" class="Slide (strict)"("Scale.Minimum"=-12.0 ("Scale.Range:Maximum")) -> ()  [unwired: 2 in, 2 out]
            n221 = property on="Sweep end" class="Slide (strict)"("Scale.Maximum"=12.0 ("Scale.Range:Maximum")) -> ()  [unwired: 2 in, 2 out]
          }
          frame "DutyCycle" {
            n222 = property on="Sweep end" class="Slide (strict)"("Scale.Minimum"=0.0 ("Scale.Range:Maximum")) -> ()  [unwired: 2 in, 2 out]
            n223 = property on="Sweep end" class="Slide (strict)"("Scale.Maximum"=100.0 ("Scale.Range:Maximum")) -> ()  [unwired: 2 in, 2 out]
            n224 = property on="Sweep start" class="Slide (strict)"("Scale.Minimum"=0.0 ("Scale.Range:Maximum")) -> ()  [unwired: 2 in, 2 out]
            n225 = property on="Sweep start" class="Slide (strict)"("Scale.Maximum"=100.0 ("Scale.Range:Maximum")) -> ()  [unwired: 2 in, 2 out]
          }
          frame "Amplitude" {
            n226 = property on="Sweep end" class="Slide (strict)"("Scale.Minimum"=0.0 ("Scale.Range:Maximum")) -> ()  [unwired: 2 in, 2 out]
            n227 = property on="Sweep start" class="Slide (strict)"("Scale.Minimum"=0.0 ("Scale.Range:Maximum")) -> ()  [unwired: 2 in, 2 out]
            n228 = property on="Sweep end" class="Slide (strict)"("Scale.Maximum"=24.0 ("Scale.Range:Maximum")) -> ()  [unwired: 2 in, 2 out]
            n229 = property on="Sweep start" class="Slide (strict)"("Scale.Maximum"=24.0 ("Scale.Range:Maximum")) -> ()  [unwired: 2 in, 2 out]
          }
        }
      }
      event "Channel A.Sweep start": Value Change {
        n230 = event-data() -> ()  [unwired: 1 in, 3 out]
        n231 = property on="Sweep start" class="Slide (strict)"() -> ("Scale.Minimum"=w467:dbl)  [unwired: 2 in, 2 out]
        n232 = Equal?(x=w467, y=-12.0) -> (x = y?=w465:bool)
        n233 = case shown="False" w465 {
          tunnel: w464 -> [w470 w487]
          tunnel: w463 -> [w471 w486]
          tunnel: [w469 w485] -> w462
          tunnel: [w468 w484] -> w461
          frame False {
            n234 = local read "Channel A"() -> (w478:T3)
            n235 = Unbundle By Name(w478) -> ("Sweep start"=w472:dbl)
            n236 = Number To Fractional String(use system decimal point (T)=FALSE, number=w472, width (-)=i16 9, precision (6)=i16 3) -> (F-format string=w480:string)
            n237 = Concatenate Strings("SST" ("string"), w480, "\n") -> (w479:string)
            n238 = VISA Write(VISA resource name=w471, write buffer=w479, error in (no error)=w470) -> (VISA resource name out=w468:refnum<visa-resource-name>, error out=w469:errorcluster)  [unwired: 1 out]
          }
          frame True {
            n239 = local read "Channel A"() -> (w493:T3)
            n240 = Unbundle By Name(w493) -> ("Sweep start"=w483:dbl)
            n241 = Add(x=w483, y=12.0) -> (x+y=w482:dbl)
            n242 = Number To Fractional String(use system decimal point (T)=FALSE, number=w482, width (-)=i16 9, precision (6)=i16 3) -> (F-format string=w495:string)
            n243 = Concatenate Strings("SST" ("string"), w495, "\n") -> (w494:string)
            n244 = VISA Write(VISA resource name=w486, write buffer=w494, error in (no error)=w487) -> (VISA resource name out=w484:refnum<visa-resource-name>, error out=w485:errorcluster)  [unwired: 1 out]
          }
        }
      }
      event "Channel A.Sweep end": Value Change {
        n245 = event-data() -> ()  [unwired: 1 in, 3 out]
        n246 = property on="Sweep end" class="Slide (strict)"() -> ("Scale.Minimum"=w502:dbl)  [unwired: 2 in, 2 out]
        n247 = Equal?(x=w502, y=-12.0) -> (x = y?=w501:bool)
        n248 = case shown="True" w501 {
          tunnel: w498 -> [w505 w522]
          tunnel: w499 -> [w506 w521]
          tunnel: [w504 w520] -> w496
          tunnel: [w503 w519] -> w497
          frame False {
            n249 = local read "Channel A"() -> (w513:T3)
            n250 = Unbundle By Name(w513) -> ("Sweep end"=w507:dbl)
            n251 = Number To Fractional String(use system decimal point (T)=FALSE, number=w507, width (-)=i16 9, precision (6)=i16 3) -> (F-format string=w515:string)
            n252 = Concatenate Strings("SEN" ("string"), w515, "\n") -> (w514:string)
            n253 = VISA Write(VISA resource name=w506, write buffer=w514, error in (no error)=w505) -> (VISA resource name out=w503:refnum<visa-resource-name>, error out=w504:errorcluster)  [unwired: 1 out]
          }
          frame True {
            n254 = local read "Channel A"() -> (w528:T3)
            n255 = Unbundle By Name(w528) -> ("Sweep end"=w518:dbl)
            n256 = Add(x=w518, y=12.0) -> (x+y=w517:dbl)
            n257 = Number To Fractional String(use system decimal point (T)=FALSE, number=w517, width (-)=i16 9, precision (6)=i16 3) -> (F-format string=w530:string)
            n258 = Concatenate Strings("SEN" ("string"), w530, "\n") -> (w529:string)
            n259 = VISA Write(VISA resource name=w521, write buffer=w529, error in (no error)=w522) -> (VISA resource name out=w519:refnum<visa-resource-name>, error out=w520:errorcluster)  [unwired: 1 out]
          }
        }
      }
      event "Channel B.Frequence": Value Change {
        n260 = event-data() -> ()  [unwired: 1 in, 3 out]
        n261 = local read "Channel B"() -> (w543:T2)
        n262 = Unbundle By Name(w543) -> ("Frequence"=w534:dbl)
        n263 = Number To Fractional String(use system decimal point (T)=FALSE, number=w534, width (-)=i16 0, precision (6)=i16 6) -> (F-format string=w542:string)
        n264 = Concatenate Strings("WFF" ("string"), w542, "\n") -> (w541:string)
        n265 = VISA Write(VISA resource name=w538, write buffer=w541, error in (no error)=w537) -> (VISA resource name out=w536:refnum<visa-resource-name>, error out=w535:errorcluster)  [unwired: 1 out]
      }
      event "Channel A.Frequence": Value Change {
        n266 = event-data() -> ()  [unwired: 1 in, 3 out]
        n267 = local read "Channel A"() -> (w552:T3)
        n268 = Unbundle By Name(w552) -> ("Frequence"=w548:dbl)
        n269 = Number To Fractional String(use system decimal point (T)=FALSE, number=w548, width (-)=i16 0, precision (6)=i16 6) -> (F-format string=w547:string)
        n270 = Concatenate Strings("WMF" ("string"), w547, "\n") -> (w549:string)
        n271 = VISA Write(VISA resource name=w556, write buffer=w549, error in (no error)=w555) -> (VISA resource name out=w554:refnum<visa-resource-name>, error out=w553:errorcluster)  [unwired: 1 out]
      }
      event "Channel A.Incr": Value Change {
        n272 = event-data() -> ()  [unwired: 1 in, 3 out]
        n273 = local read "Channel A"() -> (w558:T3)
        n274 = Unbundle By Name(w558) -> ("Incr"=w557:T13)
        n275 = case shown="\"10Mhz\"" w557 {
          frame "1uHz", Default {
            n276 = property on="Frequence" class="Knob (strict)"("Increment"=1e-06 ("Scale.Range:Increment")) -> ()  [unwired: 2 in, 2 out]
          }
          frame "10uHz" {
            n277 = property on="Frequence" class="Knob (strict)"("Increment"=1e-05 ("Scale.Range:Increment")) -> ()  [unwired: 2 in, 2 out]
          }
          frame "100uHz" {
            n278 = property on="Frequence" class="Knob (strict)"("Increment"=0.0001 ("Scale.Range:Increment")) -> ()  [unwired: 2 in, 2 out]
          }
          frame "1mHz" {
            n279 = property on="Frequence" class="Knob (strict)"("Increment"=0.001 ("Scale.Range:Increment")) -> ()  [unwired: 2 in, 2 out]
          }
          frame "10mHz" {
            n280 = property on="Frequence" class="Knob (strict)"("Increment"=0.01 ("Scale.Range:Increment")) -> ()  [unwired: 2 in, 2 out]
          }
          frame "100mHz" {
            n281 = property on="Frequence" class="Knob (strict)"("Increment"=0.1 ("Scale.Range:Increment")) -> ()  [unwired: 2 in, 2 out]
          }
          frame "1Hz" {
            n282 = property on="Frequence" class="Knob (strict)"("Increment"=1.0 ("Scale.Range:Increment")) -> ()  [unwired: 2 in, 2 out]
          }
          frame "10Hz" {
            n283 = property on="Frequence" class="Knob (strict)"("Increment"=10.0 ("Scale.Range:Increment")) -> ()  [unwired: 2 in, 2 out]
          }
          frame "100Hz" {
            n284 = property on="Frequence" class="Knob (strict)"("Increment"=100.0 ("Scale.Range:Increment")) -> ()  [unwired: 2 in, 2 out]
          }
          frame "1Khz" {
            n285 = property on="Frequence" class="Knob (strict)"("Increment"=1000.0 ("Scale.Range:Increment")) -> ()  [unwired: 2 in, 2 out]
          }
          frame "10Khz" {
            n286 = property on="Frequence" class="Knob (strict)"("Increment"=10000.0 ("Scale.Range:Increment")) -> ()  [unwired: 2 in, 2 out]
          }
          frame "100Khz" {
            n287 = property on="Frequence" class="Knob (strict)"("Increment"=100000.0 ("Scale.Range:Increment")) -> ()  [unwired: 2 in, 2 out]
          }
          frame "1Mhz" {
            n288 = property on="Frequence" class="Knob (strict)"("Increment"=1000000.0 ("Scale.Range:Increment")) -> ()  [unwired: 2 in, 2 out]
          }
          frame "10Mhz" {
            n289 = property on="Frequence" class="Knob (strict)"("Increment"=10000000.0 ("Scale.Range:Increment")) -> ()  [unwired: 2 in, 2 out]
          }
        }
      }
      event "Channel B.Incr": Value Change {
        n290 = event-data() -> ()  [unwired: 1 in, 3 out]
        n291 = local read "Channel B"() -> (w574:T2)
        n292 = Unbundle By Name(w574) -> ("Incr"=w573:T13)
        n293 = case shown="\"10Hz\"" w573 {
          frame "1uHz", Default {
            n294 = property on="Frequence" class="Knob (strict)"("Increment"=1e-06 ("Scale.Range:Increment")) -> ()  [unwired: 2 in, 2 out]
          }
          frame "10uHz" {
            n295 = property on="Frequence" class="Knob (strict)"("Increment"=1e-05 ("Scale.Range:Increment")) -> ()  [unwired: 2 in, 2 out]
          }
          frame "100uHz" {
            n296 = property on="Frequence" class="Knob (strict)"("Increment"=0.0001 ("Scale.Range:Increment")) -> ()  [unwired: 2 in, 2 out]
          }
          frame "1mHz" {
            n297 = property on="Frequence" class="Knob (strict)"("Increment"=0.001 ("Scale.Range:Increment")) -> ()  [unwired: 2 in, 2 out]
          }
          frame "10mHz" {
            n298 = property on="Frequence" class="Knob (strict)"("Increment"=0.01 ("Scale.Range:Increment")) -> ()  [unwired: 2 in, 2 out]
          }
          frame "100mHz" {
            n299 = property on="Frequence" class="Knob (strict)"("Increment"=0.1 ("Scale.Range:Increment")) -> ()  [unwired: 2 in, 2 out]
          }
          frame "1Hz" {
            n300 = property on="Frequence" class="Knob (strict)"("Increment"=1.0 ("Scale.Range:Increment")) -> ()  [unwired: 2 in, 2 out]
          }
          frame "10Hz" {
            n301 = property on="Frequence" class="Knob (strict)"("Increment"=10.0 ("Scale.Range:Increment")) -> ()  [unwired: 2 in, 2 out]
          }
          frame "100Hz" {
            n302 = property on="Frequence" class="Knob (strict)"("Increment"=100.0 ("Scale.Range:Increment")) -> ()  [unwired: 2 in, 2 out]
          }
          frame "1Khz" {
            n303 = property on="Frequence" class="Knob (strict)"("Increment"=1000.0 ("Scale.Range:Increment")) -> ()  [unwired: 2 in, 2 out]
          }
          frame "10Khz" {
            n304 = property on="Frequence" class="Knob (strict)"("Increment"=10000.0 ("Scale.Range:Increment")) -> ()  [unwired: 2 in, 2 out]
          }
          frame "100Khz" {
            n305 = property on="Frequence" class="Knob (strict)"("Increment"=100000.0 ("Scale.Range:Increment")) -> ()  [unwired: 2 in, 2 out]
          }
          frame "1Mhz" {
            n306 = property on="Frequence" class="Knob (strict)"("Increment"=1000000.0 ("Scale.Range:Increment")) -> ()  [unwired: 2 in, 2 out]
          }
          frame "10Mhz" {
            n307 = property on="Frequence" class="Knob (strict)"("Increment"=10000000.0 ("Scale.Range:Increment")) -> ()  [unwired: 2 in, 2 out]
          }
        }
      }
      event "Channel A.Incr FSK": Value Change {
        n308 = event-data() -> ()  [unwired: 1 in, 3 out]
        n309 = local read "Channel A"() -> (w590:T3)
        n310 = Unbundle By Name(w590) -> ("Incr FSK"=w589:T13)
        n311 = case shown="\"10Hz\"" w589 {
          frame "1uHz", Default {
            n312 = property on="FSK frequence" class="Knob (strict)"("Increment"=1e-06 ("Scale.Range:Increment")) -> ()  [unwired: 2 in, 2 out]
          }
          frame "10uHz" {
            n313 = property on="FSK frequence" class="Knob (strict)"("Increment"=1e-05 ("Scale.Range:Increment")) -> ()  [unwired: 2 in, 2 out]
          }
          frame "100uHz" {
            n314 = property on="FSK frequence" class="Knob (strict)"("Increment"=0.0001 ("Scale.Range:Increment")) -> ()  [unwired: 2 in, 2 out]
          }
          frame "1mHz" {
            n315 = property on="FSK frequence" class="Knob (strict)"("Increment"=0.001 ("Scale.Range:Increment")) -> ()  [unwired: 2 in, 2 out]
          }
          frame "10mHz" {
            n316 = property on="FSK frequence" class="Knob (strict)"("Increment"=0.01 ("Scale.Range:Increment")) -> ()  [unwired: 2 in, 2 out]
          }
          frame "100mHz" {
            n317 = property on="FSK frequence" class="Knob (strict)"("Increment"=0.1 ("Scale.Range:Increment")) -> ()  [unwired: 2 in, 2 out]
          }
          frame "1Hz" {
            n318 = property on="FSK frequence" class="Knob (strict)"("Increment"=1.0 ("Scale.Range:Increment")) -> ()  [unwired: 2 in, 2 out]
          }
          frame "10Hz" {
            n319 = property on="FSK frequence" class="Knob (strict)"("Increment"=10.0 ("Scale.Range:Increment")) -> ()  [unwired: 2 in, 2 out]
          }
          frame "100Hz" {
            n320 = property on="FSK frequence" class="Knob (strict)"("Increment"=100.0 ("Scale.Range:Increment")) -> ()  [unwired: 2 in, 2 out]
          }
          frame "1Khz" {
            n321 = property on="FSK frequence" class="Knob (strict)"("Increment"=1000.0 ("Scale.Range:Increment")) -> ()  [unwired: 2 in, 2 out]
          }
          frame "10Khz" {
            n322 = property on="FSK frequence" class="Knob (strict)"("Increment"=10000.0 ("Scale.Range:Increment")) -> ()  [unwired: 2 in, 2 out]
          }
          frame "100Khz" {
            n323 = property on="FSK frequence" class="Knob (strict)"("Increment"=100000.0 ("Scale.Range:Increment")) -> ()  [unwired: 2 in, 2 out]
          }
          frame "1Mhz" {
            n324 = property on="FSK frequence" class="Knob (strict)"("Increment"=1000000.0 ("Scale.Range:Increment")) -> ()  [unwired: 2 in, 2 out]
          }
          frame "10Mhz" {
            n325 = property on="FSK frequence" class="Knob (strict)"("Increment"=10000000.0 ("Scale.Range:Increment")) -> ()  [unwired: 2 in, 2 out]
          }
        }
      }
      event "Channel A.Incr Trigger": Value Change {
        n326 = event-data() -> ()  [unwired: 1 in, 3 out]
        n327 = local read "Channel A"() -> (w606:T3)
        n328 = Unbundle By Name(w606) -> ("Incr Trigger"=w605:T14)
        n329 = case shown="\"1m\"" w605 {
          frame "1u", Default {
            n330 = property on="Trigger Pulse" class="Knob (strict)"("Increment"=1e-06 ("Scale.Range:Increment")) -> ()  [unwired: 2 in, 2 out]
          }
          frame "10u" {
            n331 = property on="Trigger Pulse" class="Knob (strict)"("Increment"=1e-05 ("Scale.Range:Increment")) -> ()  [unwired: 2 in, 2 out]
          }
          frame "100u" {
            n332 = property on="Trigger Pulse" class="Knob (strict)"("Increment"=0.0001 ("Scale.Range:Increment")) -> ()  [unwired: 2 in, 2 out]
          }
          frame "1m" {
            n333 = property on="Trigger Pulse" class="Knob (strict)"("Increment"=0.001 ("Scale.Range:Increment")) -> ()  [unwired: 2 in, 2 out]
          }
          frame "10m" {
            n334 = property on="Trigger Pulse" class="Knob (strict)"("Increment"=0.01 ("Scale.Range:Increment")) -> ()  [unwired: 2 in, 2 out]
          }
          frame "100m" {
            n335 = property on="Trigger Pulse" class="Knob (strict)"("Increment"=0.1 ("Scale.Range:Increment")) -> ()  [unwired: 2 in, 2 out]
          }
          frame "1" {
            n336 = property on="Trigger Pulse" class="Knob (strict)"("Increment"=1.0 ("Scale.Range:Increment")) -> ()  [unwired: 2 in, 2 out]
          }
          frame "10" {
            n337 = property on="Trigger Pulse" class="Knob (strict)"("Increment"=10.0 ("Scale.Range:Increment")) -> ()  [unwired: 2 in, 2 out]
          }
          frame "100" {
            n338 = property on="Trigger Pulse" class="Knob (strict)"("Increment"=100.0 ("Scale.Range:Increment")) -> ()  [unwired: 2 in, 2 out]
          }
          frame "1K" {
            n339 = property on="Trigger Pulse" class="Knob (strict)"("Increment"=1000.0 ("Scale.Range:Increment")) -> ()  [unwired: 2 in, 2 out]
          }
          frame "10K" {
            n340 = property on="Trigger Pulse" class="Knob (strict)"("Increment"=10000.0 ("Scale.Range:Increment")) -> ()  [unwired: 2 in, 2 out]
          }
          frame "100K" {
            n341 = property on="Trigger Pulse" class="Knob (strict)"("Increment"=100000.0 ("Scale.Range:Increment")) -> ()  [unwired: 2 in, 2 out]
          }
        }
      }
      event "Channel A.Incr FM": Value Change {
        n342 = event-data() -> ()  [unwired: 1 in, 3 out]
        n343 = local read "Channel A"() -> (w620:T3)
        n344 = Unbundle By Name(w620) -> ("Incr FM"=w619:T13)
        n345 = case shown="\"10Mhz\"" w619 {
          frame "1uHz", Default {
            n346 = property on="FM Freq offset" class="Slide (strict)"("Increment"=1e-06 ("Scale.Range:Increment")) -> ()  [unwired: 2 in, 2 out]
          }
          frame "10uHz" {
            n347 = property on="FM Freq offset" class="Slide (strict)"("Increment"=1e-05 ("Scale.Range:Increment")) -> ()  [unwired: 2 in, 2 out]
          }
          frame "100uHz" {
            n348 = property on="FM Freq offset" class="Slide (strict)"("Increment"=0.0001 ("Scale.Range:Increment")) -> ()  [unwired: 2 in, 2 out]
          }
          frame "1mHz" {
            n349 = property on="FM Freq offset" class="Slide (strict)"("Increment"=0.001 ("Scale.Range:Increment")) -> ()  [unwired: 2 in, 2 out]
          }
          frame "10mHz" {
            n350 = property on="FM Freq offset" class="Slide (strict)"("Increment"=0.01 ("Scale.Range:Increment")) -> ()  [unwired: 2 in, 2 out]
          }
          frame "100mHz" {
            n351 = property on="FM Freq offset" class="Slide (strict)"("Increment"=0.1 ("Scale.Range:Increment")) -> ()  [unwired: 2 in, 2 out]
          }
          frame "1Hz" {
            n352 = property on="FM Freq offset" class="Slide (strict)"("Increment"=1.0 ("Scale.Range:Increment")) -> ()  [unwired: 2 in, 2 out]
          }
          frame "10Hz" {
            n353 = property on="FM Freq offset" class="Slide (strict)"("Increment"=10.0 ("Scale.Range:Increment")) -> ()  [unwired: 2 in, 2 out]
          }
          frame "100Hz" {
            n354 = property on="FM Freq offset" class="Slide (strict)"("Increment"=100.0 ("Scale.Range:Increment")) -> ()  [unwired: 2 in, 2 out]
          }
          frame "1Khz" {
            n355 = property on="FM Freq offset" class="Slide (strict)"("Increment"=1000.0 ("Scale.Range:Increment")) -> ()  [unwired: 2 in, 2 out]
          }
          frame "10Khz" {
            n356 = property on="FM Freq offset" class="Slide (strict)"("Increment"=10000.0 ("Scale.Range:Increment")) -> ()  [unwired: 2 in, 2 out]
          }
          frame "100Khz" {
            n357 = property on="FM Freq offset" class="Slide (strict)"("Increment"=100000.0 ("Scale.Range:Increment")) -> ()  [unwired: 2 in, 2 out]
          }
          frame "1Mhz" {
            n358 = property on="FM Freq offset" class="Slide (strict)"("Increment"=1000000.0 ("Scale.Range:Increment")) -> ()  [unwired: 2 in, 2 out]
          }
          frame "10Mhz" {
            n359 = property on="FM Freq offset" class="Slide (strict)"("Increment"=10000000.0 ("Scale.Range:Increment")) -> ()  [unwired: 2 in, 2 out]
          }
        }
      }
      event "Channel A.Offset": Value Change {
        n360 = event-data() -> ()  [unwired: 1 in, 3 out]
        n361 = local read "Channel A"() -> (w647:T3)
        n362 = Unbundle By Name(w647) -> ("Offset"=w639:dbl)
        n363 = Number To Fractional String(use system decimal point (T)=FALSE, number=w639, width (-)=i16 5, precision (6)=i16 4 ("width (-)")) -> (F-format string=w637:string)
        n364 = Concatenate Strings("WMO" ("string"), w637, "\n") -> (w641:string)
        n365 = VISA Write(VISA resource name=w646, write buffer=w641, error in (no error)=w645) -> (VISA resource name out=w644:refnum<visa-resource-name>, error out=w643:errorcluster)  [unwired: 1 out]
      }
      event "Channel A.Phase": Value Change {
        n366 = event-data() -> ()  [unwired: 1 in, 3 out]
        n367 = local read "Channel A"() -> (w660:T3)
        n368 = Unbundle By Name(w660) -> ("Phase"=w652:dbl)
        n369 = Number To Fractional String(use system decimal point (T)=FALSE, number=w652, width (-)=i16 6, precision (6)=i16 3) -> (F-format string=w651:string)
        n370 = Concatenate Strings("WMP" ("string"), w651, "\n") -> (w654:string)
        n371 = VISA Write(VISA resource name=w659, write buffer=w654, error in (no error)=w658) -> (VISA resource name out=w657:refnum<visa-resource-name>, error out=w656:errorcluster)  [unwired: 1 out]
      }
      event "stop": Value Change {
        n372 = event-data() -> ()  [unwired: 1 in, 3 out]
      }
      event "Channel A.DutyCycle": Value Change {
        n373 = event-data() -> ()  [unwired: 1 in, 3 out]
        n374 = local read "Channel A"() -> (w676:T3)
        n375 = Unbundle By Name(w676) -> ("DutyCycle"=w668:dbl)
        n376 = Number To Fractional String(use system decimal point (T)=FALSE, number=w668, width (-)=i16 6, precision (6)=i16 3) -> (F-format string=w667:string)
        n377 = Concatenate Strings("WMD" ("string"), w667, "\n") -> (w670:string)
        n378 = VISA Write(VISA resource name=w675, write buffer=w670, error in (no error)=w674) -> (VISA resource name out=w673:refnum<visa-resource-name>, error out=w672:errorcluster)  [unwired: 1 out]
      }
    }
  }
  n379 = VISA Close(VISA resource name=w48, error in (no error)=w47) -> ()  [unwired: 1 out]
